vi "WriteConfigKeys.vi"(0 "GRMActor in":refnum<class "GenericController.lvclass">, 1 "StringValues":string[](array[string]), 5 "Config Refnum":T1, 7 "Keys":string[](array[string]), 9 "DoubleValue":dbl[](array[numeric]), 11 "error in (no error)":errorcluster, 12 "BoolValues":bool[](array[boolean])) -> (4 "GRMActor out":refnum<class "GenericController.lvclass">, 6 "Config Refnum dup":T1, 15 "error out":errorcluster)   [LabVIEW 2020, in "GenericController.lvlib" / "GenericController.lvclass"]
uses:
  GenericController.lvclass
  <vilib>/Utility/config.llb/Config Data RefNum.ctl
  <vilib>/Utility/config.llb/Write Key (String).vi
  <vilib>/Utility/config.llb/Write Key (Boolean).vi
  <vilib>/Utility/config.llb/Write Key (Double).vi
  <vilib>/Utility/config.llb/NI_LVConfig.lvlib
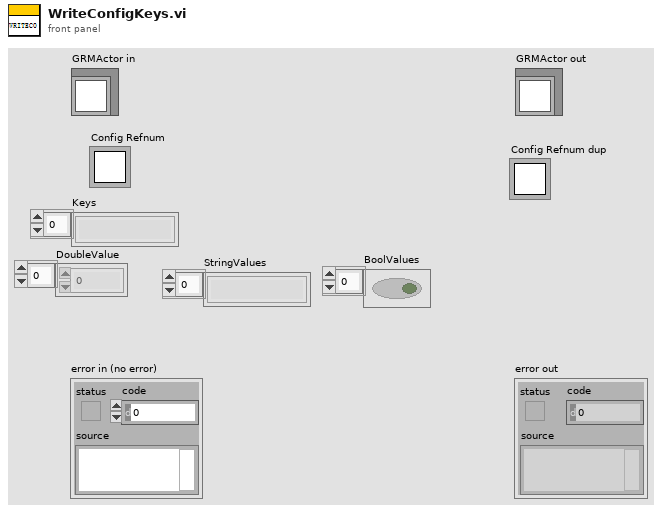
[diagram p1: front panel]
types:
  T1 = typedef "NI_LVConfig.lvlib/Config Data RefNum.ctl" = refnum<k1>
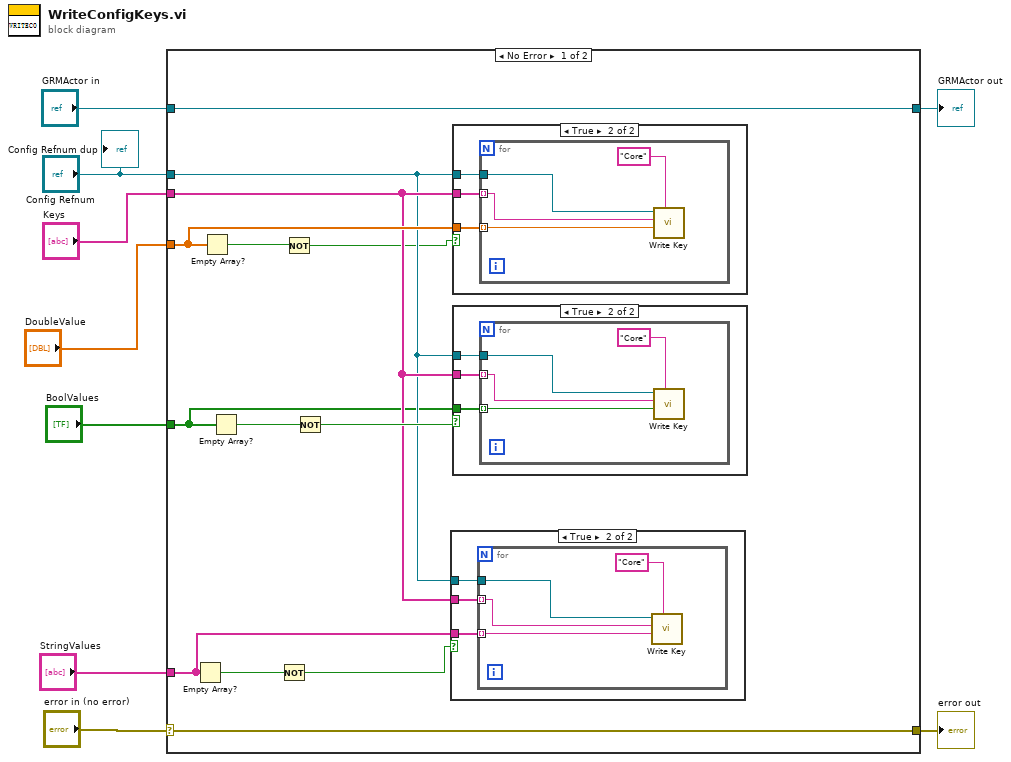
[diagram p0: block diagram]
diagram:
  n1 = case shown="No Error" "error in (no error)" {
    selector: "error in (no error)" -> [w21 w45]
    tunnel: [w21 w45] -> w8
    tunnel: [w22 w44] -> w6
    tunnel: "GRMActor in" -> [w22 w44]
    tunnel: "Config Refnum" -> [w12 _]
    tunnel: "Keys" -> [w13 _]
    tunnel: "DoubleValue" -> [w20 _]
    tunnel: "BoolValues" -> [w11 _]
    tunnel: "StringValues" -> [w15 _]
    frame No Error {
      n2 = Empty Array?(array=w15) -> (empty?=w17:bool)
      n3 = Empty Array?(array=w20) -> (empty?=w19:bool)
      n4 = Empty Array?(array=w11) -> (empty?=w18:bool)
      n5 = Not(x=w17) -> (.not. x?=w16:bool)
      n6 = Not(x=w19) -> (.not. x?=w10:bool)
      n7 = Not(x=w18) -> (.not. x?=w14:bool)
      n8 = case shown="True" w16 {
        tunnel: w12 -> [_ w25]
        tunnel: w13 -> [_ w24]
        tunnel: w15 -> [_ w23]
        frame False {
        }
        frame True {
          n9 = for {
            tunnel: w25 -> [w28]
            tunnel: w24 -> [w27] mode=indexing
            tunnel: w23 -> [w26] mode=indexing
            n10 = call-poly <vilib>:"Write Key.vi"("section"="Core", "value"=w26, "key"=w27, "refnum"=w28) -> ()  [unwired: 5 in, 3 out]
          }
        }
      }
      n11 = case shown="True" w10 {
        tunnel: w12 -> [_ w39]
        tunnel: w13 -> [_ w38]
        tunnel: w20 -> [_ w37]
        frame False {
        }
        frame True {
          n12 = for {
            tunnel: w39 -> [w42]
            tunnel: w38 -> [w41] mode=indexing
            tunnel: w37 -> [w40] mode=indexing
            n13 = call-poly <vilib>:"Write Key.vi"("section"="Core", "value"=w40, "key"=w41, "refnum"=w42) -> ()  [unwired: 5 in, 3 out]
          }
        }
      }
      n14 = case shown="True" w14 {
        tunnel: w12 -> [_ w32]
        tunnel: w13 -> [_ w31]
        tunnel: w11 -> [_ w30]
        frame False {
        }
        frame True {
          n15 = for {
            tunnel: w32 -> [w35]
            tunnel: w31 -> [w34] mode=indexing
            tunnel: w30 -> [w33] mode=indexing
            n16 = call-poly <vilib>:"Write Key.vi"("section"="Core", "value"=w33, "key"=w34, "refnum"=w35) -> ()  [unwired: 5 in, 3 out]
          }
        }
      }
    }
    frame Error {
    }
  }
  "error out" <- w8
  "GRMActor out" <- w6
  "Config Refnum dup" <- "Config Refnum"
